vi "Cache Panel Blank.vi"(8 "error in (no error)":errorcluster, 11 "2DArrayManager in":refnum<class "2DArrayManager.lvclass">) -> (0 "error out":errorcluster, 3 "2DArrayManager out":refnum<class "2DArrayManager.lvclass">)   [LabVIEW 2020, in "OOPanel.lvlib" / "2DArrayManager.lvclass"]
uses:
  2DArrayManager.lvclass
  ArrayPanel/ArrayPanel.lvclass
  2DArrayManager.lvclass/2DArrayManager.ctl
  2DPanelBlank/2DPanelBlank.lvclass
  C:/dev/lv20CE/lv-oopanel/OOPanel/ArrayPanel/ArrayPanel.lvclass
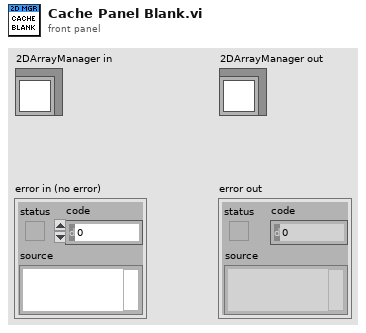
[diagram p1: front panel]
types:
  T1 = typedef "OOPanel.lvlib/2DArrayManager.lvclass/Options.ctl" = cluster{"Running":bool, "Borders":bool, "Background":u32, "V Scroll":bool, "H Scroll":bool, "Blank":refnum<class "2DPanelBlank.lvclass">}
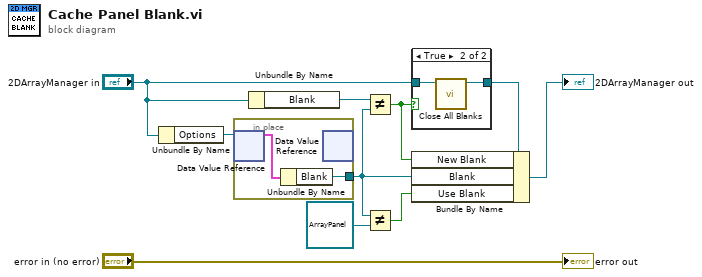
[diagram p0: block diagram]
diagram:
  n1 = Unbundle By Name("2DArrayManager in") -> ("Options"=w9:refnum<data-value>)
  n2 = in-place {
    in-place-border: [w11] -> w5
    n3 = in-place-dvr #1(w9) -> (w12:T1)  [unwired: 1 out]
    n4 = Unbundle By Name(w12) -> ("Blank"=w11:refnum<class "2DPanelBlank.lvclass">)
    n5 = in-place-dvr #1() -> ()  [unwired: 1 in, 2 out]
  }
  n6 = Unbundle By Name("2DArrayManager in") -> ("Blank"=w4:refnum<class "2DPanelBlank.lvclass">)
  n7 = Not Equal?(x=w4, y=w5) -> (x != y?=w2:bool)
  n8 = Not Equal?(x=w5, y=refnum<class "ArrayPanel.lvclass"> refnum) -> (x != y?=w8:bool)
  n9 = case shown="True" w2 {
    tunnel: "2DArrayManager in" -> [w13 w15]
    tunnel: [w13 w14] -> w3
    frame False {
    }
    frame True {
      n10 = call "Close All Blanks.vi"("2DArrayManager in"=w15) -> ("2DArrayManager out"=w14:refnum<class "2DArrayManager.lvclass">)  [unwired: 9 in, 1 out]
    }
  }
  n11 = Bundle By Name(cluster=w3, "New Blank"=w2, "Blank"=w5, "Use Blank"=w8) -> (→"2DArrayManager out":refnum<class "2DArrayManager.lvclass">)
  "error out" <- "error in (no error)"
